vi "AlGaInPAs_prep_run_cont_dil_v10.vi"(2 "Debug Mode":bool, 3 "Elapsed Time(s)":dbl, 4 "State":enum16{"Edit", "Start", "Run", "End", "Idle"}(ring), 5 "Argument List In":string[](array[string])) -> (0 "Status Out":string, 1 "Argument List Out":string[](array[string]))   [LabVIEW 2011]
panel:
  out "Prep-In var":bool
  out "Prep-Ga var":bool
  out "Prep-Al var":bool
  out "Prep-P var":bool
  out "Prep-As var":bool
  out "prep_done":bool
  out "run started":bool
  out "first":bool=TRUE
  out "total time":dbl
  out "is OK?":bool
  out "AsH3?":bool
  out "PH3?":bool
  out "In?":bool
  out "Ga?":bool
  out "Al?":bool
  in  "Prep As":bool caption="Pre-run"
  in  "Prep P":bool caption="Pre-run"
  in  "Prep In":bool caption="Pre-run"
  in  "prep_time":dbl caption="pre-run time (s)"
  in  "Prep Al":bool caption="Pre-run"
  in  "Run As":bool caption="Run"
  in  "AsH3 Flow":dbl caption="AsH3 Flow (0-10 sccm)" format="%.2f"
  in  "P Flow":dbl caption="P Flow (0-100 sccm)" format="%.2f"
  in  "Run P":bool caption="Run"
  in  "In Flow":dbl caption="In Flow (0-100 sscm)" format="%.2f"
  in  "Run In":bool caption="Run"
  in  "Run Al":bool caption="Run"
  in  "Al Flow":dbl caption="Al Flow (0-100 sscm)" format="%.2f"
  in  "Cancel":bool
  in  "OK":bool
  out "tTotal(s) 2":dbl
  in  "Ga Tab Control":enum32{"Page 1", "Page 2"}(tab)
  in  "Ga Dilution":bool caption="Dilute"
  in  "Ga Flow":dbl caption="Ga Flow (0-10 sscm)" format="%.4f"
  in  "Run Ga":bool caption="Run"
  in  "Prep Ga":bool caption="Pre-run"
  in  "GAMFC1":dbl=1.0 caption="R1 (0-10 sscm)" format="%.2f"
  out "GAMFC2 set":dbl caption="R2 (0-100 sscm)" format="%.2f"
  in  "GAMFC3":dbl=100.0 caption="R3 (0-1000 sscm)" format="%.1f"
  out "GAMFC1 set":dbl caption="R1 (0-10 sscm)" format="%.2f"
  # "Add pre-run time to run time in editor."
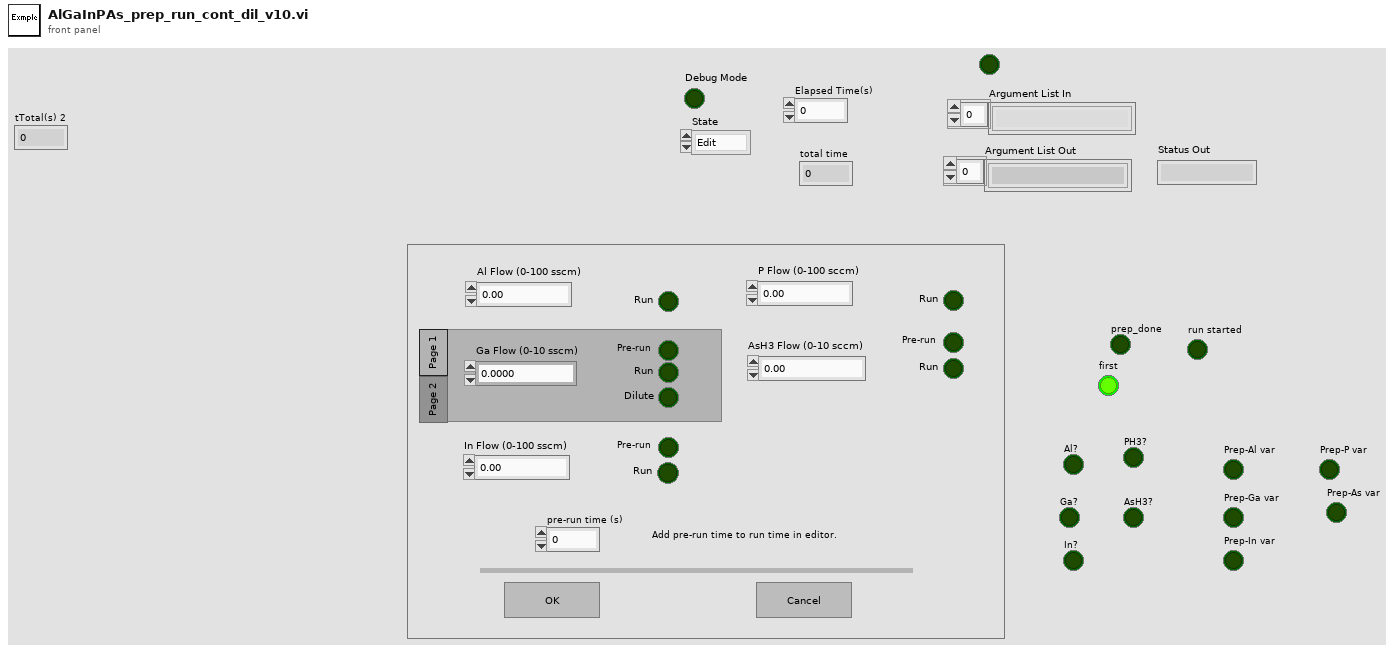
[diagram p1: front panel]
types:
  T1 = enum16{"Discrete", "Continuous", "Instantaneous", "Finite"}
  T2 = enum32{"Invalid", "Default", "Floating", "Floating/Auto-Hide", "Modal"}
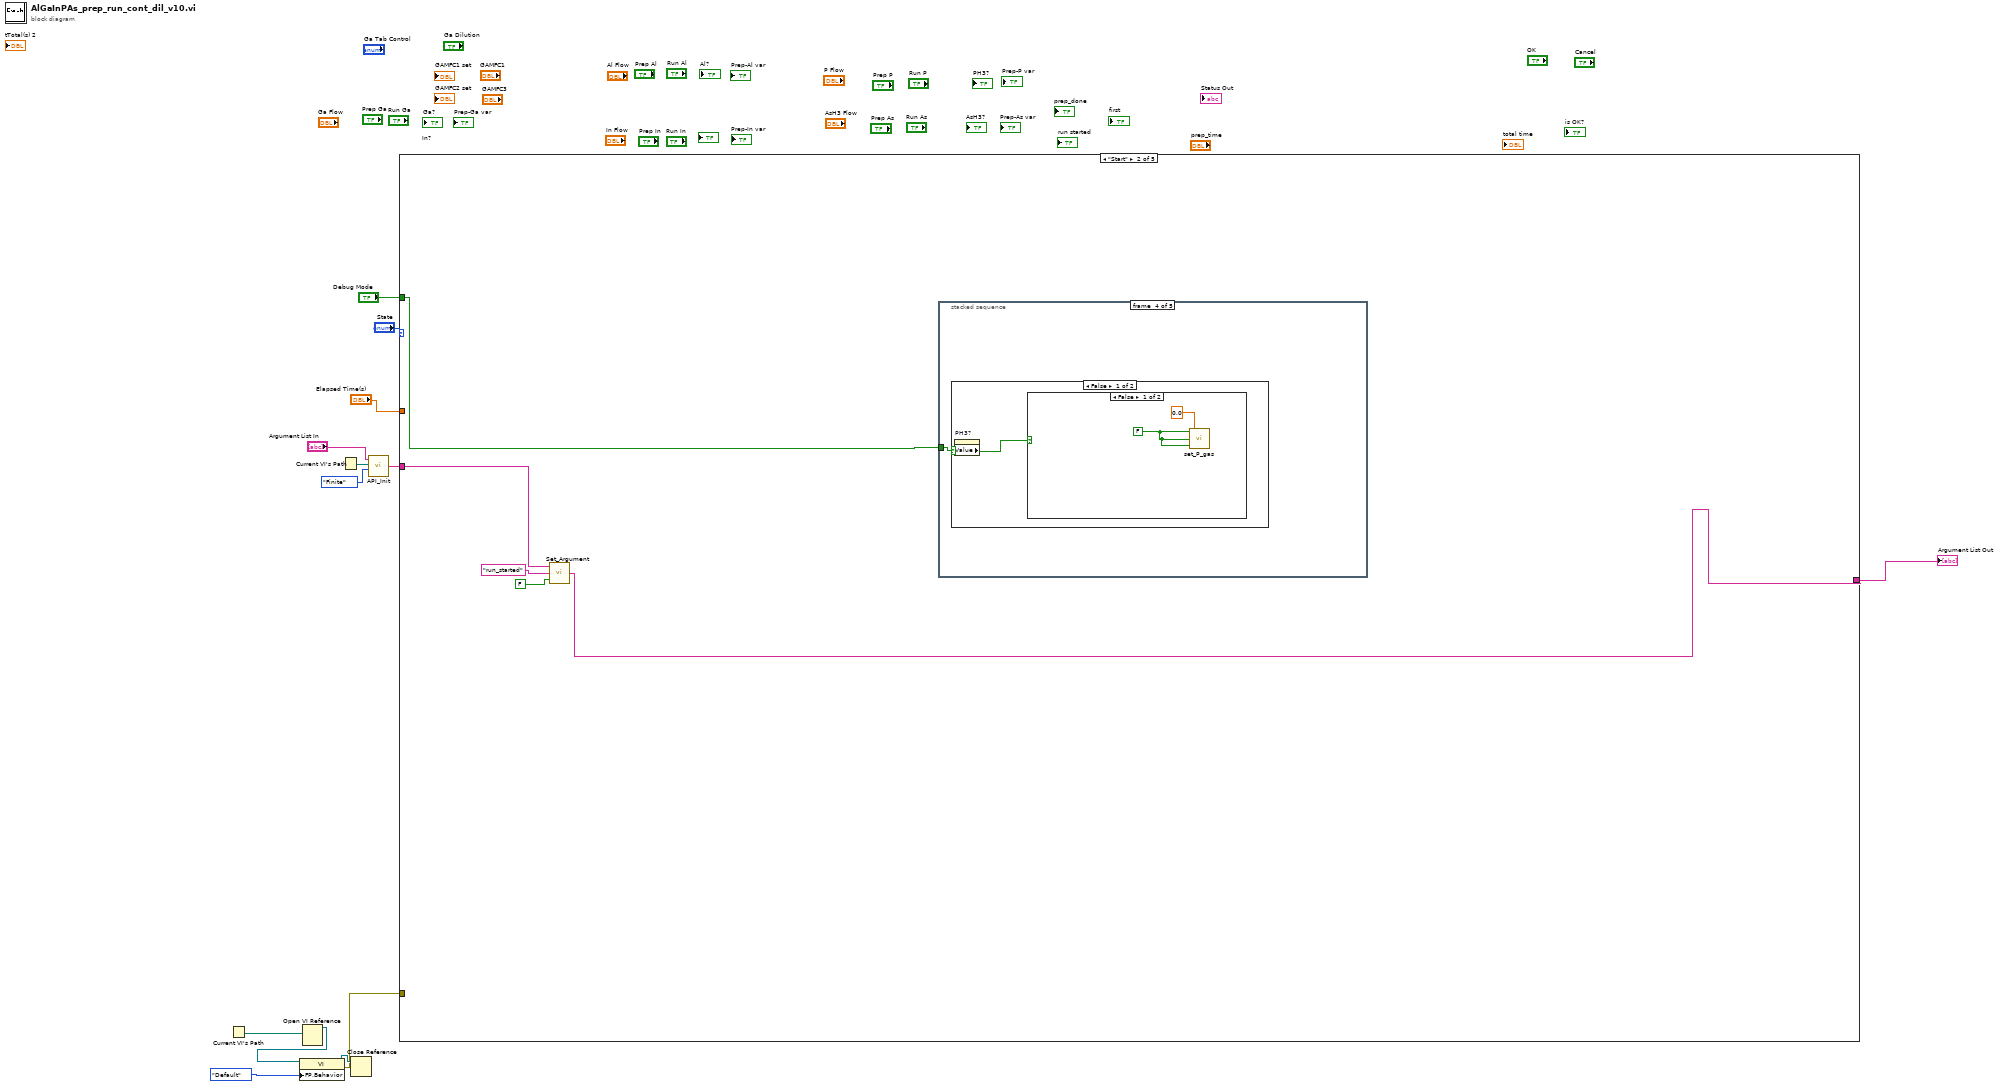
[diagram p0: block diagram]
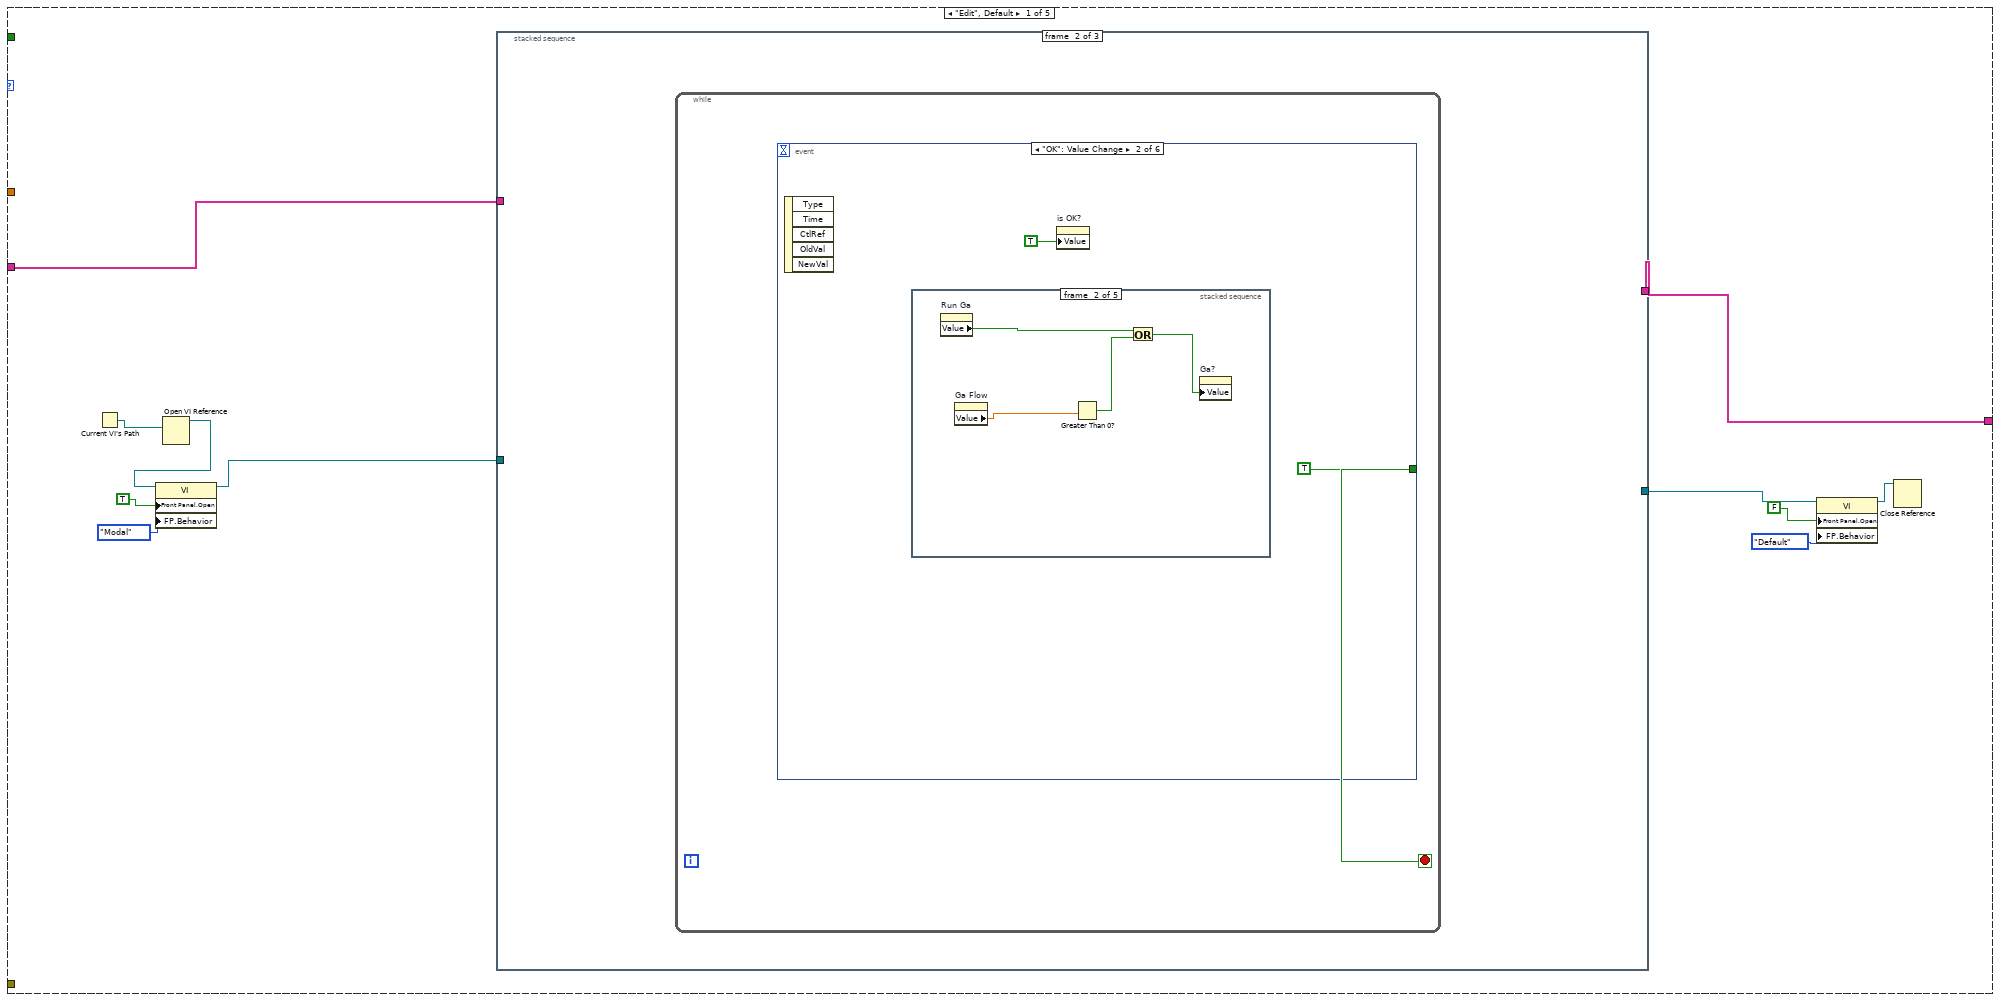
[diagram p2: hidden frame]
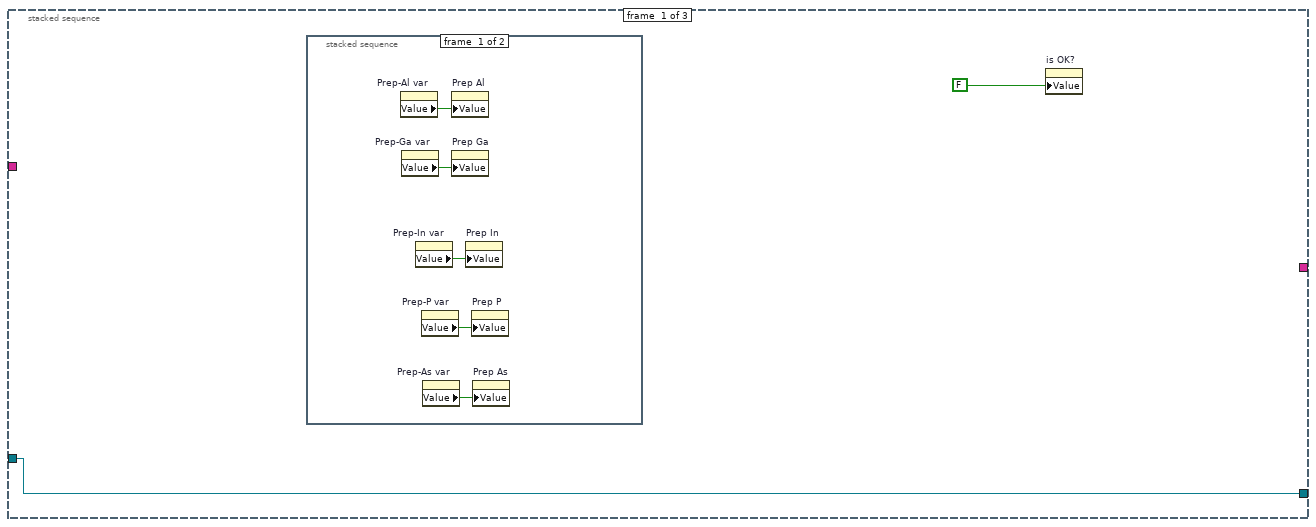
[diagram p3: hidden frame]
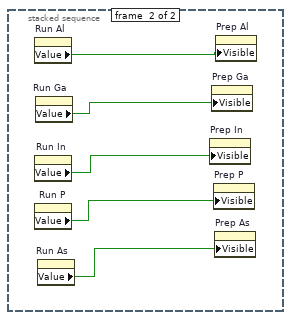
[diagram p4: hidden frame]
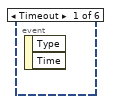
[diagram p5: hidden frame]
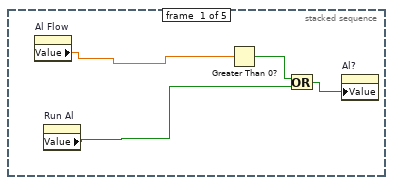
[diagram p6: hidden frame]
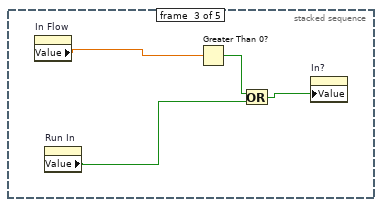
[diagram p7: hidden frame]
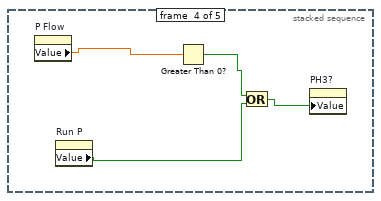
[diagram p8: hidden frame]
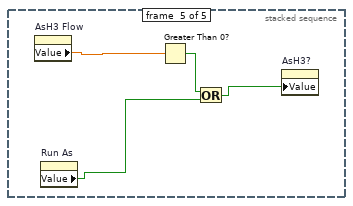
[diagram p9: hidden frame]
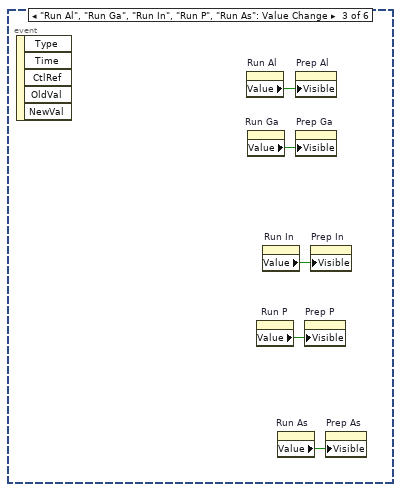
[diagram p10: hidden frame]
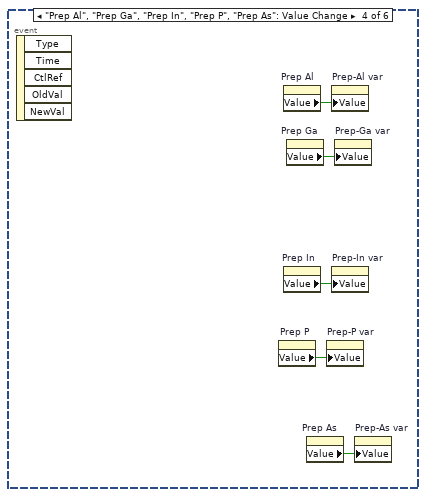
[diagram p11: hidden frame]
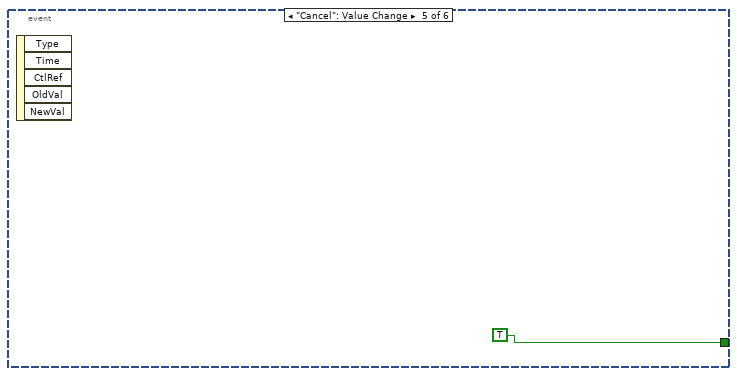
[diagram p12: hidden frame]
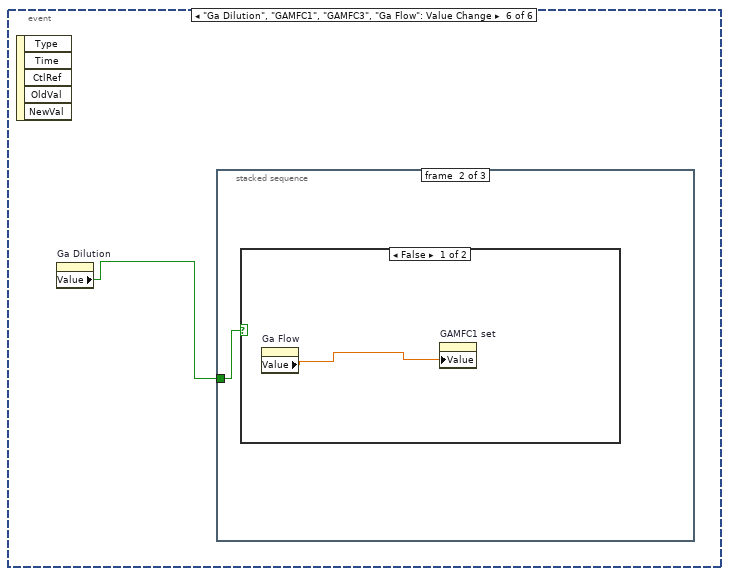
[diagram p13: hidden frame]
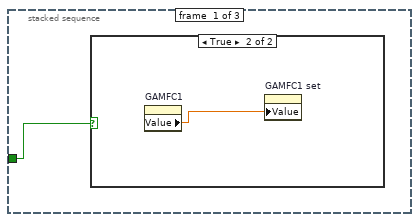
[diagram p14: hidden frame]
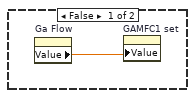
[diagram p15: hidden frame]
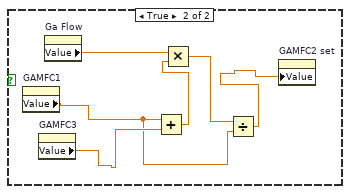
[diagram p16: hidden frame]
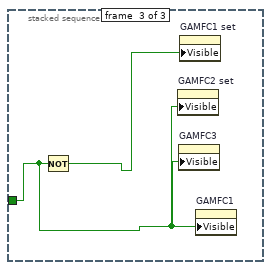
[diagram p17: hidden frame]
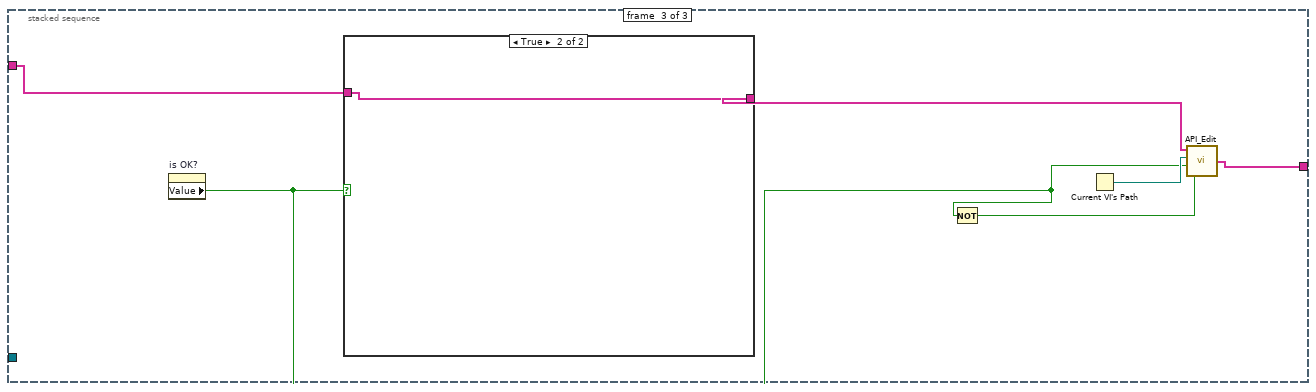
[diagram p18: hidden frame]
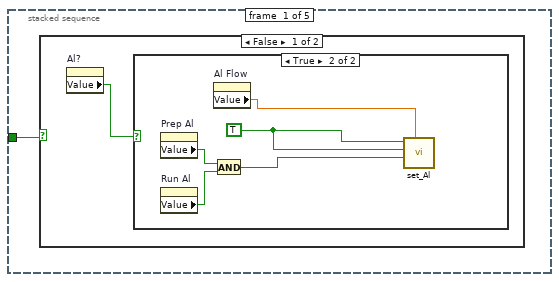
[diagram p20: hidden frame]
diagram:
  n1 = Current VI's Path() -> (path=w9:path)
  n2 = Open VI Reference(vi path=w9) -> (vi reference=w8:refnum<vi>)  [unwired: 1 in, 5 out]
  n3 = property class="VI"(reference=w8, "FP.Behavior"=T2."Default" ("Front Panel Window:Behavior")) -> (reference out=w6:refnum<vi>, error out=w5:errorcluster)  [unwired: 1 in]
  n4 = Current VI's Path() -> (path=w4:path)
  n5 = Close Reference(reference=w6) -> ()  [unwired: 1 in, 1 out]
  n6 = call "API_Init.vi"("API Mode"=T1."Finite", "VI Path"=w4, "Argument List In"="Argument List In") -> ("Argument List Out"=w1:string[])  [unwired: 1 in]
  n7 = case shown="\"Start\"" "State" {
    tunnel: "Debug Mode" -> [_ w93 w150 _ _]
    tunnel: "Elapsed Time(s)" -> [_ _ w152 _ _]
    tunnel: w1 -> [w15 w95 w149 w269 w270]
    tunnel: [w14 w94 w151 w269 w270] -> w10
    tunnel: w5 -> [_ _ _ _ _]
    frame "Edit", Default {
      n8 = Current VI's Path() -> (path=w20:path)
      n9 = Open VI Reference(vi path=w20) -> (vi reference=w19:refnum<vi>)  [unwired: 1 in, 5 out]
      n10 = property class="VI"(reference=w19, "Front Panel.Open"=TRUE ("Front Panel Window:Open"), "FP.Behavior"=T2."Modal" ("Front Panel Window:Behavior")) -> (reference out=w18:refnum<vi>)  [unwired: 1 in, 1 out]
      n11 = stacked-sequence {
        tunnel: w15 -> [_ _ w88]
        tunnel: w18 -> [w26 _ _]
        tunnel: [w26 _ _] -> w22
        tunnel: [_ _ w86] -> w14
        frame #0 {
          n12 = stacked-sequence {
            frame #0 {
              n13 = property on="Prep-Al var" class="Bool (strict)"() -> ("Value"=w31:bool)  [unwired: 2 in, 2 out]
              n14 = property on="Prep-Ga var" class="Bool (strict)"() -> ("Value"=w30:bool)  [unwired: 2 in, 2 out]
              n15 = property on="Prep-In var" class="Bool (strict)"() -> ("Value"=w29:bool)  [unwired: 2 in, 2 out]
              n16 = property on="Prep-P var" class="Bool (strict)"() -> ("Value"=w28:bool)  [unwired: 2 in, 2 out]
              n17 = property on="Prep-As var" class="Bool (strict)"() -> ("Value"=w27:bool)  [unwired: 2 in, 2 out]
              n18 = property on="Prep Al" class="Bool (strict)"("Value"=w31) -> ()  [unwired: 2 in, 2 out]
              n19 = property on="Prep Ga" class="Bool (strict)"("Value"=w30) -> ()  [unwired: 2 in, 2 out]
              n20 = property on="Prep In" class="Bool (strict)"("Value"=w29) -> ()  [unwired: 2 in, 2 out]
              n21 = property on="Prep P" class="Bool (strict)"("Value"=w28) -> ()  [unwired: 2 in, 2 out]
              n22 = property on="Prep As" class="Bool (strict)"("Value"=w27) -> ()  [unwired: 2 in, 2 out]
            }
            frame #1 {
              n23 = property on="Run Al" class="Bool (strict)"() -> ("Value"=w36:bool)  [unwired: 2 in, 2 out]
              n24 = property on="Run In" class="Bool (strict)"() -> ("Value"=w34:bool)  [unwired: 2 in, 2 out]
              n25 = property on="Run P" class="Bool (strict)"() -> ("Value"=w33:bool)  [unwired: 2 in, 2 out]
              n26 = property on="Run Ga" class="Bool (strict)"() -> ("Value"=w35:bool)  [unwired: 2 in, 2 out]
              n27 = property on="Run As" class="Bool (strict)"() -> ("Value"=w32:bool)  [unwired: 2 in, 2 out]
              n28 = property on="Prep In" class="Bool (strict)"("Visible"=w34) -> ()  [unwired: 2 in, 2 out]
              n29 = property on="Prep Ga" class="Bool (strict)"("Visible"=w35) -> ()  [unwired: 2 in, 2 out]
              n30 = property on="Prep P" class="Bool (strict)"("Visible"=w33) -> ()  [unwired: 2 in, 2 out]
              n31 = property on="Prep As" class="Bool (strict)"("Visible"=w32) -> ()  [unwired: 2 in, 2 out]
              n32 = property on="Prep Al" class="Bool (strict)"("Visible"=w36) -> ()  [unwired: 2 in, 2 out]
            }
          }
          n33 = property on="is OK?" class="Bool (strict)"("Value"=FALSE ("is OK?")) -> ()  [unwired: 2 in, 2 out]
        }
        frame #1 {
          n34 = while {
            stop <- w37 stop-if-true
            n35 = event shown="[1] \"OK\": Value Change" {
              selector: _ -> [_ _ _ _ _ _]
              dyn-events: _ -> [_ _ _ _ _ _]
              timeout: _ -> [_ _ _ _ _ _]
              tunnel: [_ TRUE _ _ TRUE _] -> w37
              event Timeout {
                n36 = event-data() -> ()  [unwired: 1 in, 2 out]
              }
              event "OK": Value Change {
                n37 = event-data() -> ()  [unwired: 1 in, 5 out]
                n38 = stacked-sequence {
                  frame #0 {
                    n39 = property on="Al Flow" class="DigNum (strict)"() -> ("Value"=w42:dbl)  [unwired: 2 in, 2 out]
                    n40 = property on="Run Al" class="Bool (strict)"() -> ("Value"=w41:bool)  [unwired: 2 in, 2 out]
                    n41 = Greater Than 0?(x=w42) -> (x > 0?=w43:bool)
                    n42 = Or(x=w43, y=w41) -> (x .or. y?=w40:bool)
                    n43 = property on="Al?" class="Bool (strict)"("Value"=w40) -> ()  [unwired: 2 in, 2 out]
                  }
                  frame #1 {
                    n44 = property on="Run Ga" class="Bool (strict)"() -> ("Value"=w45:bool)  [unwired: 2 in, 2 out]
                    n45 = property on="Ga Flow" class="DigNum (strict)"() -> ("Value"=w46:dbl)  [unwired: 2 in, 2 out]
                    n46 = Greater Than 0?(x=w46) -> (x > 0?=w47:bool)
                    n47 = Or(x=w45, y=w47) -> (x .or. y?=w44:bool)
                    n48 = property on="Ga?" class="Bool (strict)"("Value"=w44) -> ()  [unwired: 2 in, 2 out]
                  }
                  frame #2 {
                    n49 = property on="In Flow" class="DigNum (strict)"() -> ("Value"=w49:dbl)  [unwired: 2 in, 2 out]
                    n50 = property on="Run In" class="Bool (strict)"() -> ("Value"=w50:bool)  [unwired: 2 in, 2 out]
                    n51 = Greater Than 0?(x=w49) -> (x > 0?=w51:bool)
                    n52 = Or(x=w51, y=w50) -> (x .or. y?=w48:bool)
                    n53 = property on="In?" class="Bool (strict)"("Value"=w48) -> ()  [unwired: 2 in, 2 out]
                  }
                  frame #3 {
                    n54 = property on="P Flow" class="DigNum (strict)"() -> ("Value"=w54:dbl)  [unwired: 2 in, 2 out]
                    n55 = property on="Run P" class="Bool (strict)"() -> ("Value"=w53:bool)  [unwired: 2 in, 2 out]
                    n56 = Greater Than 0?(x=w54) -> (x > 0?=w55:bool)
                    n57 = Or(x=w55, y=w53) -> (x .or. y?=w52:bool)
                    n58 = property on="PH3?" class="Bool (strict)"("Value"=w52) -> ()  [unwired: 2 in, 2 out]
                  }
                  frame #4 {
                    n59 = property on="AsH3 Flow" class="DigNum (strict)"() -> ("Value"=w58:dbl)  [unwired: 2 in, 2 out]
                    n60 = property on="Run As" class="Bool (strict)"() -> ("Value"=w57:bool)  [unwired: 2 in, 2 out]
                    n61 = Greater Than 0?(x=w58) -> (x > 0?=w59:bool)
                    n62 = Or(x=w59, y=w57) -> (x .or. y?=w56:bool)
                    n63 = property on="AsH3?" class="Bool (strict)"("Value"=w56) -> ()  [unwired: 2 in, 2 out]
                  }
                }
                n64 = property on="is OK?" class="Bool (strict)"("Value"=TRUE ("is OK?")) -> ()  [unwired: 2 in, 2 out]
              }
              event "Run Al", "Run Ga", "Run In", "Run P", "Run As": Value Change {
                n65 = event-data() -> ()  [unwired: 1 in, 5 out]
                n66 = property on="Run Al" class="Bool (strict)"() -> ("Value"=w64:bool)  [unwired: 2 in, 2 out]
                n67 = property on="Run Ga" class="Bool (strict)"() -> ("Value"=w63:bool)  [unwired: 2 in, 2 out]
                n68 = property on="Run P" class="Bool (strict)"() -> ("Value"=w60:bool)  [unwired: 2 in, 2 out]
                n69 = property on="Run In" class="Bool (strict)"() -> ("Value"=w62:bool)  [unwired: 2 in, 2 out]
                n70 = property on="Run As" class="Bool (strict)"() -> ("Value"=w61:bool)  [unwired: 2 in, 2 out]
                n71 = property on="Prep Al" class="Bool (strict)"("Visible"=w64) -> ()  [unwired: 2 in, 2 out]
                n72 = property on="Prep Ga" class="Bool (strict)"("Visible"=w63) -> ()  [unwired: 2 in, 2 out]
                n73 = property on="Prep P" class="Bool (strict)"("Visible"=w60) -> ()  [unwired: 2 in, 2 out]
                n74 = property on="Prep In" class="Bool (strict)"("Visible"=w62) -> ()  [unwired: 2 in, 2 out]
                n75 = property on="Prep As" class="Bool (strict)"("Visible"=w61) -> ()  [unwired: 2 in, 2 out]
              }
              event "Prep Al", "Prep Ga", "Prep In", "Prep P", "Prep As": Value Change {
                n76 = event-data() -> ()  [unwired: 1 in, 5 out]
                n77 = property on="Prep P" class="Bool (strict)"() -> ("Value"=w66:bool)  [unwired: 2 in, 2 out]
                n78 = property on="Prep Al" class="Bool (strict)"() -> ("Value"=w69:bool)  [unwired: 2 in, 2 out]
                n79 = property on="Prep In" class="Bool (strict)"() -> ("Value"=w67:bool)  [unwired: 2 in, 2 out]
                n80 = property on="Prep Ga" class="Bool (strict)"() -> ("Value"=w68:bool)  [unwired: 2 in, 2 out]
                n81 = property on="Prep As" class="Bool (strict)"() -> ("Value"=w65:bool)  [unwired: 2 in, 2 out]
                n82 = property on="Prep-P var" class="Bool (strict)"("Value"=w66) -> ()  [unwired: 2 in, 2 out]
                n83 = property on="Prep-Al var" class="Bool (strict)"("Value"=w69) -> ()  [unwired: 2 in, 2 out]
                n84 = property on="Prep-In var" class="Bool (strict)"("Value"=w67) -> ()  [unwired: 2 in, 2 out]
                n85 = property on="Prep-Ga var" class="Bool (strict)"("Value"=w68) -> ()  [unwired: 2 in, 2 out]
                n86 = property on="Prep-As var" class="Bool (strict)"("Value"=w65) -> ()  [unwired: 2 in, 2 out]
              }
              event "Cancel": Value Change {
                n87 = event-data() -> ()  [unwired: 1 in, 5 out]
              }
              event "Ga Dilution", "GAMFC1", "GAMFC3", "Ga Flow": Value Change {
                n88 = event-data() -> ()  [unwired: 1 in, 5 out]
                n89 = property on="Ga Dilution" class="Bool (strict)"() -> ("Value"=w71:bool)  [unwired: 2 in, 2 out]
                n90 = stacked-sequence {
                  tunnel: w71 -> [w72 w75 w83]
                  frame #0 {
                    n91 = case shown="True" w72 {
                      frame False {
                        n92 = property on="Ga Flow" class="DigNum (strict)"() -> ("Value"=w73:dbl)  [unwired: 2 in, 2 out]
                        n93 = property on="GAMFC1 set" class="DigNum (strict)"("Value"=w73) -> ()  [unwired: 2 in, 2 out]
                      }
                      frame True {
                        n94 = property on="GAMFC1" class="DigNum (strict)"() -> ("Value"=w74:dbl)  [unwired: 2 in, 2 out]
                        n95 = property on="GAMFC1 set" class="DigNum (strict)"("Value"=w74) -> ()  [unwired: 2 in, 2 out]
                      }
                    }
                  }
                  frame #1 {
                    n96 = case shown="False" w75 {
                      frame False {
                        n97 = property on="Ga Flow" class="DigNum (strict)"() -> ("Value"=w76:dbl)  [unwired: 2 in, 2 out]
                        n98 = property on="GAMFC1 set" class="DigNum (strict)"("Value"=w76) -> ()  [unwired: 2 in, 2 out]
                      }
                      frame True {
                        n99 = property on="GAMFC1" class="DigNum (strict)"() -> ("Value"=w77:dbl)  [unwired: 2 in, 2 out]
                        n100 = property on="GAMFC3" class="DigNum (strict)"() -> ("Value"=w79:dbl)  [unwired: 2 in, 2 out]
                        n101 = property on="Ga Flow" class="DigNum (strict)"() -> ("Value"=w80:dbl)  [unwired: 2 in, 2 out]
                        n102 = Add(x=w77, y=w79) -> (x+y=w82:dbl)
                        n103 = Multiply(x=w80, y=w82) -> (x*y=w78:dbl)
                        n104 = Divide(x=w78, y=w77) -> (x/y=w81:dbl)
                        n105 = property on="GAMFC2 set" class="DigNum (strict)"("Value"=w81) -> ()  [unwired: 2 in, 2 out]
                      }
                    }
                  }
                  frame #2 {
                    n106 = Not(x=w83) -> (.not. x?=w84:bool)
                    n107 = property on="GAMFC2 set" class="DigNum (strict)"("Visible"=w83) -> ()  [unwired: 2 in, 2 out]
                    n108 = property on="GAMFC3" class="DigNum (strict)"("Visible"=w83) -> ()  [unwired: 2 in, 2 out]
                    n109 = property on="GAMFC1 set" class="DigNum (strict)"("Visible"=w84) -> ()  [unwired: 2 in, 2 out]
                    n110 = property on="GAMFC1" class="DigNum (strict)"("Visible"=w83) -> ()  [unwired: 2 in, 2 out]
                  }
                }
              }
            }
          }
        }
        frame #2 {
          n111 = property on="is OK?" class="Bool (strict)"() -> ("Value"=w85:bool)  [unwired: 2 in, 2 out]
          n112 = case shown="True" w85 {
            tunnel: w88 -> [w91 w92]
            tunnel: [w91 w92] -> w87
            frame False {
            }
            frame True {
            }
          }
          n113 = Not(x=w85) -> (.not. x?=w90:bool)
          n114 = Current VI's Path() -> (path=w89:path)
          n115 = call "API_Edit.vi"("Cancel"=w90, "OK"=w85, "VI Path"=w89, "Argument List In"=w87) -> ("Argument List Out"=w86:string[])
        }
      }
      n116 = property class="VI"(reference=w22, "Front Panel.Open"=FALSE ("Front Panel Window:Open"), "FP.Behavior"=T2."Default" ("Front Panel Window:Behavior")) -> (reference out=w23:refnum<vi>)  [unwired: 1 in, 1 out]
      n117 = Close Reference(reference=w23) -> ()  [unwired: 1 in, 1 out]
    }
    frame "Start" {
      n118 = call "Set_Argument.vi"("Enable"=FALSE, "Argument"="run_started", "Argument List In"=w95) -> ("Argument List Out"=w94:string[])
      n119 = stacked-sequence {
        tunnel: w93 -> [w98 w107 w122 w131 w140]
        frame #0 {
          n120 = case shown="False" w98 {
            frame False {
              n121 = property on="Al?" class="Bool (strict)"() -> ("Value"=w99:bool)  [unwired: 2 in, 2 out]
              n122 = case shown="True" w99 {
                frame False {
                  w100 = FALSE ("Al Active")
                  n123 = call "set_Al.vi"("ALMFC1"=0.0 ("Aluminum Flow"), "Remote"=w100, "Run"=w100, "Bubbler In"=w100, "Active"=w100) -> ()  [unwired: 5 out]
                }
                frame True {
                  w106 = TRUE ("Al Active")
                  n124 = property on="Prep Al" class="Bool (strict)"() -> ("Value"=w104:bool)  [unwired: 2 in, 2 out]
                  n125 = property on="Run Al" class="Bool (strict)"() -> ("Value"=w103:bool)  [unwired: 2 in, 2 out]
                  n126 = property on="Al Flow" class="DigNum (strict)"() -> ("Value"=w105:dbl)  [unwired: 2 in, 2 out]
                  n127 = And(x=w104, y=w103) -> (x .and. y?=w102:bool)
                  n128 = call "set_Al.vi"("ALMFC1"=w105, "Run"=w102, "Bubbler In"=w106, "Active"=w106) -> ()  [unwired: 1 in, 5 out]
                }
              }
            }
            frame True {
            }
          }
        }
        frame #1 {
          n129 = case shown="False" w107 {
            frame False {
              n130 = property on="Ga?" class="Bool (strict)"() -> ("Value"=w108:bool)  [unwired: 2 in, 2 out]
              n131 = case shown="True" w108 {
                frame False {
                  w110 = FALSE ("Ga Active")
                  w109 = 0.0 ("Ga Flow 1")
                  n132 = call "set_Ga.vi"("Active"=w110, "GAMFC3"=w109, "GAMFC2"=w109, "GAMFC1"=w109, "Bubbler In"=w110, "H2 Dilute"=w110, "Run"=w110, "Remote"=w110) -> ()  [unwired: 8 out]
                }
                frame True {
                  w113 = TRUE ("Ga Active")
                  n133 = property on="Ga Dilution" class="Bool (strict)"() -> ("Value"=w112:bool)  [unwired: 2 in, 2 out]
                  n134 = property on="GAMFC2 set" class="DigNum (strict)"() -> ("Value"=w115:dbl)  [unwired: 2 in, 2 out]
                  n135 = property on="GAMFC3" class="DigNum (strict)"() -> ("Value"=w114:dbl)  [unwired: 2 in, 2 out]
                  n136 = property on="Prep-Ga var" class="Bool (strict)"() -> ("Value"=w116:bool)  [unwired: 2 in, 2 out]
                  n137 = property on="Run Ga" class="Bool (strict)"() -> ("Value"=w117:bool)  [unwired: 2 in, 2 out]
                  n138 = case shown="True" w112 {
                    tunnel: [w120 w121] -> w111
                    frame False {
                      n139 = property on="GAMFC1 set" class="DigNum (strict)"() -> ("Value"=w120:dbl)  [unwired: 2 in, 2 out]
                    }
                    frame True {
                      n140 = property on="GAMFC1" class="DigNum (strict)"() -> ("Value"=w121:dbl)  [unwired: 2 in, 2 out]
                    }
                  }
                  n141 = And(x=w116, y=w117) -> (x .and. y?=w119:bool)
                  n142 = property on="Ga Dilution" class="Bool (strict)"() -> ("Value"=w118:bool)  [unwired: 2 in, 2 out]
                  n143 = call "set_Ga.vi"("Active"=w113, "GAMFC3"=w114, "GAMFC2"=w115, "GAMFC1"=w111, "Bubbler In"=w113, "H2 Dilute"=w118, "Run"=w119, "Remote"=w113) -> ()  [unwired: 8 in]
                }
              }
            }
            frame True {
            }
          }
        }
        frame #2 {
          n144 = case shown="False" w122 {
            frame False {
              n145 = property on="In?" class="Bool (strict)"() -> ("Value"=w123:bool)  [unwired: 2 in, 2 out]
              n146 = case shown="True" w123 {
                frame False {
                  w125 = FALSE ("In Remote")
                  n147 = call "set_In.vi"("INMFC1"=0.0 ("Indium Flow"), "Remote"=w125, "Run"=w125, "Bubbler In"=w125, "Active"=w125) -> ()  [unwired: 5 out]
                }
                frame True {
                  w130 = TRUE ("In Run")
                  n148 = property on="Run In" class="Bool (strict)"() -> ("Value"=w127:bool)  [unwired: 2 in, 2 out]
                  n149 = property on="Prep In" class="Bool (strict)"() -> ("Value"=w128:bool)  [unwired: 2 in, 2 out]
                  n150 = And(x=w128, y=w127) -> (x .and. y?=w126:bool)
                  n151 = property on="In Flow" class="DigNum (strict)"() -> ("Value"=w129:dbl)  [unwired: 2 in, 2 out]
                  n152 = call "set_In.vi"("INMFC1"=w129, "Run"=w126, "Bubbler In"=w130, "Active"=w130) -> ()  [unwired: 1 in, 5 out]
                }
              }
            }
            frame True {
            }
          }
        }
        frame #3 {
          n153 = case shown="False" w131 {
            frame False {
              n154 = property on="PH3?" class="Bool (strict)"() -> ("Value"=w132:bool)  [unwired: 2 in, 2 out]
              n155 = case shown="False" w132 {
                frame False {
                  w133 = FALSE ("P_Gas Active")
                  n156 = call "set_P_gas.vi"("Run"=w133, "Gas In"=w133, "Active"=w133, "P_Gas Remote"=w133, "H2 Flush"=w133, "P_Gas Flow"=0.0) -> ()
                }
                frame True {
                  w139 = TRUE ("P_Gas Active")
                  n157 = property on="P Flow" class="DigNum (strict)"() -> ("Value"=w138:dbl)  [unwired: 2 in, 2 out]
                  n158 = property on="Prep P" class="Bool (strict)"() -> ("Value"=w137:bool)  [unwired: 2 in, 2 out]
                  n159 = property on="Run P" class="Bool (strict)"() -> ("Value"=w136:bool)  [unwired: 2 in, 2 out]
                  n160 = And(x=w137, y=w136) -> (x .and. y?=w135:bool)
                  n161 = call "set_P_gas.vi"("Active"=w139, "P_Gas Remote"=w135, "H2 Flush"=w139, "P_Gas Flow"=w138) -> ()  [unwired: 2 in]
                }
              }
            }
            frame True {
            }
          }
        }
        frame #4 {
          n162 = case shown="False" w140 {
            frame False {
              n163 = property on="AsH3?" class="Bool (strict)"() -> ("Value"=w141:bool)  [unwired: 2 in, 2 out]
              n164 = case shown="True" w141 {
                frame False {
                  w142 = FALSE ("As_Gas Active")
                  n165 = call "set_As_gas.vi"("Active"=w142, "As_Gas Flow"=0.0, "Gas In"=w142, "H2 Flush"=w142, "Run"=w142, "Remote"=w142) -> ()  [unwired: 10 in]
                }
                frame True {
                  w148 = TRUE ("As_Gas Active")
                  n166 = property on="Prep As" class="Bool (strict)"() -> ("Value"=w145:bool)  [unwired: 2 in, 2 out]
                  n167 = property on="Run As" class="Bool (strict)"() -> ("Value"=w146:bool)  [unwired: 2 in, 2 out]
                  n168 = property on="AsH3 Flow" class="DigNum (strict)"() -> ("Value"=w147:dbl)  [unwired: 2 in, 2 out]
                  n169 = And(x=w145, y=w146) -> (x .and. y?=w144:bool)
                  n170 = call "set_As_gas.vi"("Active"=w148, "As_Gas Flow"=w147, "Gas In"=w148, "Run"=w144) -> ()  [unwired: 12 in]
                }
              }
            }
            frame True {
            }
          }
        }
      }
    }
    frame "Run" {
      n171 = stacked-sequence {
        tunnel: w152 -> [_ w157 _ _]
        tunnel: w149 -> [w154 _ _ w211]
        tunnel: [_ _ _ w210] -> w151
        tunnel: w150 -> [_ _ _ w212]
        frame #0 {
          n172 = call "Get_Argument.vi"("Argument"="run_started", "Argument List"=w154) -> ("Enabled"=w153:bool)
          n173 = local write "run started"(w153) -> ()
        }
        frame #1 {
          n174 = property on="prep_time" class="DigNum (strict)"() -> ("Value"=w158:dbl)  [unwired: 2 in, 2 out]
          n175 = Greater Or Equal?(x=w157, y=w158) -> (x >= y?=w156:bool)
          n176 = local write "prep_done"(w156) -> ()
        }
        frame #2 {
          n177 = local read "run started"() -> (w160:bool)
          n178 = Not(x=w160) -> (.not. x?=w159:bool)
          n179 = stacked-sequence {
            tunnel: w159 -> [w162 w166 w175 w184 w193 w202]
            frame #0 {
              n180 = case shown="True" w162 {
                tunnel: ["run: " "pre-run: "] -> w161
                frame False {
                }
                frame True {
                }
              }
              n181 = property on="Status Out" class="Str"("Value"=w161) -> ()  [unwired: 2 in, 2 out]
            }
            frame #1 {
              n182 = property on="Status Out" class="Str"() -> ("Value"=w172:string)  [unwired: 2 in, 2 out]
              n183 = property on="Al?" class="Bool (strict)"() -> ("Value"=w173:bool)  [unwired: 2 in, 2 out]
              n184 = property on="Run Al" class="Bool (strict)"() -> ("Value"=w165:bool)  [unwired: 2 in, 2 out]
              n185 = property on="Prep Al" class="Bool (strict)"() -> ("Value"=w167:bool)  [unwired: 2 in, 2 out]
              n186 = call "flow_strings.vi"("string in"=w172, "is first in?"=TRUE, "use source?"=w173, "name"="Al", "run source?"=w165, "prep source?"=w167, "is prep?"=w166) -> ("string out"=w171:string, "is first out?"=w170:bool)
              n187 = property on="Status Out" class="Str"("Value"=w171) -> ()  [unwired: 2 in, 2 out]
              n188 = property on="first" class="Bool (strict)"("Value"=w170) -> ()  [unwired: 2 in, 2 out]
            }
            frame #2 {
              n189 = property on="first" class="Bool (strict)"() -> ("Value"=w178:bool)  [unwired: 2 in, 2 out]
              n190 = property on="Status Out" class="Str"() -> ("Value"=w181:string)  [unwired: 2 in, 2 out]
              n191 = property on="Ga?" class="Bool (strict)"() -> ("Value"=w179:bool)  [unwired: 2 in, 2 out]
              n192 = property on="Run Ga" class="Bool (strict)"() -> ("Value"=w174:bool)  [unwired: 2 in, 2 out]
              n193 = property on="Prep Ga" class="Bool (strict)"() -> ("Value"=w176:bool)  [unwired: 2 in, 2 out]
              n194 = call "flow_strings.vi"("string in"=w181, "is first in?"=w178, "use source?"=w179, "name"="Ga", "run source?"=w174, "prep source?"=w176, "is prep?"=w175) -> ("string out"=w182:string, "is first out?"=w177:bool)
              n195 = property on="Status Out" class="Str"("Value"=w182) -> ()  [unwired: 2 in, 2 out]
              n196 = property on="first" class="Bool (strict)"("Value"=w177) -> ()  [unwired: 2 in, 2 out]
            }
            frame #3 {
              n197 = property on="first" class="Bool (strict)"() -> ("Value"=w188:bool)  [unwired: 2 in, 2 out]
              n198 = property on="Status Out" class="Str"() -> ("Value"=w190:string)  [unwired: 2 in, 2 out]
              n199 = property on="In?" class="Bool (strict)"() -> ("Value"=w191:bool)  [unwired: 2 in, 2 out]
              n200 = property on="Run In" class="Bool (strict)"() -> ("Value"=w183:bool)  [unwired: 2 in, 2 out]
              n201 = property on="Prep In" class="Bool (strict)"() -> ("Value"=w185:bool)  [unwired: 2 in, 2 out]
              n202 = call "flow_strings.vi"("string in"=w190, "is first in?"=w188, "use source?"=w191, "name"="In", "run source?"=w183, "prep source?"=w185, "is prep?"=w184) -> ("string out"=w187:string, "is first out?"=w186:bool)
              n203 = property on="Status Out" class="Str"("Value"=w187) -> ()  [unwired: 2 in, 2 out]
              n204 = property on="first" class="Bool (strict)"("Value"=w186) -> ()  [unwired: 2 in, 2 out]
            }
            frame #4 {
              n205 = property on="first" class="Bool (strict)"() -> ("Value"=w196:bool)  [unwired: 2 in, 2 out]
              n206 = property on="Status Out" class="Str"() -> ("Value"=w198:string)  [unwired: 2 in, 2 out]
              n207 = property on="PH3?" class="Bool (strict)"() -> ("Value"=w199:bool)  [unwired: 2 in, 2 out]
              n208 = property on="Run P" class="Bool (strict)"() -> ("Value"=w192:bool)  [unwired: 2 in, 2 out]
              n209 = property on="Prep P" class="Bool (strict)"() -> ("Value"=w194:bool)  [unwired: 2 in, 2 out]
              n210 = call "flow_strings.vi"("string in"=w198, "is first in?"=w196, "use source?"=w199, "name"="P", "run source?"=w192, "prep source?"=w194, "is prep?"=w193) -> ("string out"=w197:string, "is first out?"=w195:bool)
              n211 = property on="Status Out" class="Str"("Value"=w197) -> ()  [unwired: 2 in, 2 out]
              n212 = property on="first" class="Bool (strict)"("Value"=w195) -> ()  [unwired: 2 in, 2 out]
            }
            frame #5 {
              n213 = property on="first" class="Bool (strict)"() -> ("Value"=w205:bool)  [unwired: 2 in, 2 out]
              n214 = property on="Status Out" class="Str"() -> ("Value"=w207:string)  [unwired: 2 in, 2 out]
              n215 = property on="AsH3?" class="Bool (strict)"() -> ("Value"=w208:bool)  [unwired: 2 in, 2 out]
              n216 = property on="Run As" class="Bool (strict)"() -> ("Value"=w201:bool)  [unwired: 2 in, 2 out]
              n217 = property on="Prep As" class="Bool (strict)"() -> ("Value"=w203:bool)  [unwired: 2 in, 2 out]
              n218 = call "flow_strings.vi"("string in"=w207, "is first in?"=w205, "use source?"=w208, "name"="As", "run source?"=w201, "prep source?"=w203, "is prep?"=w202) -> ("string out"=w204:string, "is first out?"=w206:bool)
              n219 = property on="Status Out" class="Str"("Value"=w204) -> ()  [unwired: 2 in, 2 out]
              n220 = property on="first" class="Bool (strict)"("Value"=w206) -> ()  [unwired: 2 in, 2 out]
            }
          }
        }
        frame #3 {
          n221 = local read "run started"() -> (w215:bool)
          n222 = local read "prep_done"() -> (w213:bool)
          n223 = Not(x=w215) -> (.not. x?=w216:bool)
          n224 = And(x=w213, y=w216) -> (x .and. y?=w214:bool)
          n225 = stacked-sequence {
            tunnel: w214 -> [w220]
            tunnel: w212 -> [w219]
            tunnel: w211 -> [w218]
            tunnel: [w217] -> w210
            frame #0 {
              n226 = case shown="True" w220 {
                tunnel: w219 -> [_ w224]
                tunnel: w218 -> [w221 w223]
                tunnel: [w221 w222] -> w217
                frame False {
                }
                frame True {
                  n227 = stacked-sequence {
                    tunnel: w224 -> [w225 w232 w244 w251 w258 _]
                    tunnel: w223 -> [_ _ _ _ _ w266]
                    tunnel: [_ _ _ _ _ w265] -> w222
                    frame #0 {
                      n228 = case shown="False" w225 {
                        frame False {
                          n229 = property on="Al?" class="Bool (strict)"() -> ("Value"=w226:bool)  [unwired: 2 in, 2 out]
                          n230 = case shown="True" w226 {
                            frame False {
                              w227 = FALSE ("Al Active")
                              n231 = call "set_Al.vi"("ALMFC1"=0.0 ("Aluminum Flow"), "Remote"=w227, "Run"=w227, "Bubbler In"=w227, "Active"=w227) -> ()  [unwired: 5 out]
                            }
                            frame True {
                              w231 = TRUE ("Al Active")
                              n232 = property on="Al Flow" class="DigNum (strict)"() -> ("Value"=w230:dbl)  [unwired: 2 in, 2 out]
                              n233 = property on="Run Al" class="Bool (strict)"() -> ("Value"=w229:bool)  [unwired: 2 in, 2 out]
                              n234 = call "set_Al.vi"("ALMFC1"=w230, "Run"=w229, "Bubbler In"=w231, "Active"=w231) -> ()  [unwired: 1 in, 5 out]
                            }
                          }
                        }
                        frame True {
                        }
                      }
                    }
                    frame #1 {
                      n235 = case shown="False" w232 {
                        frame False {
                          n236 = property on="Ga?" class="Bool (strict)"() -> ("Value"=w233:bool)  [unwired: 2 in, 2 out]
                          n237 = case shown="True" w233 {
                            frame False {
                              w235 = FALSE ("Ga Active")
                              w234 = 0.0 ("Ga Flow 1")
                              n238 = call "set_Ga.vi"("Active"=w235, "GAMFC3"=w234, "GAMFC2"=w234, "GAMFC1"=w234, "Bubbler In"=w235, "H2 Dilute"=w235, "Run"=w235, "Remote"=w235) -> ()  [unwired: 8 out]
                            }
                            frame True {
                              w237 = TRUE ("Ga Active")
                              n239 = property on="Ga Dilution" class="Bool (strict)"() -> ("Value"=w236:bool)  [unwired: 2 in, 2 out]
                              n240 = property on="Run Ga" class="Bool (strict)"() -> ("Value"=w238:bool)  [unwired: 2 in, 2 out]
                              n241 = property on="GAMFC3" class="DigNum (strict)"() -> ("Value"=w239:dbl)  [unwired: 2 in, 2 out]
                              n242 = property on="GAMFC2 set" class="DigNum (strict)"() -> ("Value"=w240:dbl)  [unwired: 2 in, 2 out]
                              n243 = case shown="True" w236 {
                                tunnel: [w242 w243] -> w241
                                frame False {
                                n244 = property on="GAMFC1 set" class="DigNum (strict)"() -> ("Value"=w242:dbl)  [unwired: 2 in, 2 out]
                                }
                                frame True {
                                n245 = property on="GAMFC1" class="DigNum (strict)"() -> ("Value"=w243:dbl)  [unwired: 2 in, 2 out]
                                }
                              }
                              n246 = call "set_Ga.vi"("Active"=w237, "GAMFC3"=w239, "GAMFC2"=w240, "GAMFC1"=w241, "Bubbler In"=w237, "H2 Dilute"=w236, "Run"=w238, "Remote"=w237) -> ()  [unwired: 8 in]
                            }
                          }
                        }
                        frame True {
                        }
                      }
                    }
                    frame #2 {
                      n247 = case shown="False" w244 {
                        frame False {
                          n248 = property on="In?" class="Bool (strict)"() -> ("Value"=w245:bool)  [unwired: 2 in, 2 out]
                          n249 = case shown="True" w245 {
                            frame False {
                              w247 = FALSE ("In Remote")
                              n250 = call "set_In.vi"("INMFC1"=0.0 ("Indium Flow"), "Remote"=w247, "Run"=w247, "Bubbler In"=w247, "Active"=w247) -> ()  [unwired: 5 out]
                            }
                            frame True {
                              w250 = TRUE ("In Run")
                              n251 = property on="Run In" class="Bool (strict)"() -> ("Value"=w248:bool)  [unwired: 2 in, 2 out]
                              n252 = property on="In Flow" class="DigNum (strict)"() -> ("Value"=w249:dbl)  [unwired: 2 in, 2 out]
                              n253 = call "set_In.vi"("INMFC1"=w249, "Run"=w248, "Bubbler In"=w250, "Active"=w250) -> ()  [unwired: 1 in, 5 out]
                            }
                          }
                        }
                        frame True {
                        }
                      }
                    }
                    frame #3 {
                      n254 = case shown="False" w251 {
                        frame False {
                          n255 = property on="PH3?" class="Bool (strict)"() -> ("Value"=w252:bool)  [unwired: 2 in, 2 out]
                          n256 = case shown="True" w252 {
                            frame False {
                              w253 = FALSE ("P_Gas Active")
                              n257 = call "set_P_gas.vi"("Run"=w253, "Gas In"=w253, "Active"=w253, "P_Gas Remote"=w253, "H2 Flush"=w253, "P_Gas Flow"=0.0) -> ()
                            }
                            frame True {
                              w257 = TRUE ("P_Gas Active")
                              n258 = property on="P Flow" class="DigNum (strict)"() -> ("Value"=w256:dbl)  [unwired: 2 in, 2 out]
                              n259 = property on="Run P" class="Bool (strict)"() -> ("Value"=w255:bool)  [unwired: 2 in, 2 out]
                              n260 = call "set_P_gas.vi"("Active"=w257, "P_Gas Remote"=w255, "H2 Flush"=w257, "P_Gas Flow"=w256) -> ()  [unwired: 2 in]
                            }
                          }
                        }
                        frame True {
                        }
                      }
                    }
                    frame #4 {
                      n261 = case shown="False" w258 {
                        frame False {
                          n262 = property on="AsH3?" class="Bool (strict)"() -> ("Value"=w259:bool)  [unwired: 2 in, 2 out]
                          n263 = case shown="True" w259 {
                            frame False {
                              w260 = FALSE ("As_Gas Active")
                              n264 = call "set_As_gas.vi"("Active"=w260, "As_Gas Flow"=0.0, "Gas In"=w260, "H2 Flush"=w260, "Run"=w260, "Remote"=w260) -> ()  [unwired: 10 in]
                            }
                            frame True {
                              w263 = TRUE ("As_Gas Active")
                              n265 = property on="Run As" class="Bool (strict)"() -> ("Value"=w262:bool)  [unwired: 2 in, 2 out]
                              n266 = property on="AsH3 Flow" class="DigNum (strict)"() -> ("Value"=w264:dbl)  [unwired: 2 in, 2 out]
                              n267 = call "set_As_gas.vi"("Active"=w263, "As_Gas Flow"=w264, "Gas In"=w263, "Run"=w262) -> ()  [unwired: 12 in]
                            }
                          }
                        }
                        frame True {
                        }
                      }
                    }
                    frame #5 {
                      n268 = call "Set_Argument.vi"("Enable"=TRUE, "Argument"="run_started", "Argument List In"=w266) -> ("Argument List Out"=w265:string[])
                    }
                  }
                }
              }
            }
          }
        }
      }
    }
    frame "End" {
    }
    frame "Idle" {
    }
  }
  "Argument List Out" <- w10
